vi "Ball Intake SS Implem.vi"(11 "Ball Intake Commands Out":T1) -> (3 "Ball Intake Actuator Out":T2)   [LabVIEW 2016]
uses:
  Ball Intake Actuator Out.ctl
  Ball Intake Commands.ctl
  Ball Intake Logging Values.vi
  Global Variables/Robot Status.vi
  Global Variables/Ball Intake Calibrations.vi
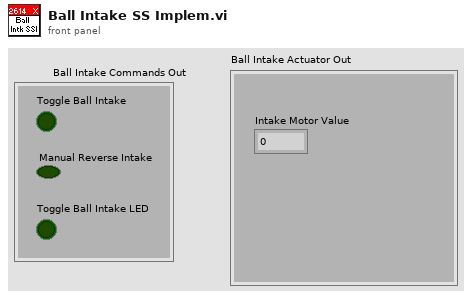
[diagram p1: front panel]
types:
  T1 = typedef "Ball Intake Commands.ctl" = cluster{"Toggle Ball Intake":bool, "Manual Reverse Intake":bool, "Toggle Ball Intake LED":bool}
  T2 = typedef "Ball Intake Actuator Out.ctl" = cluster{"Intake Motor Value":dbl}
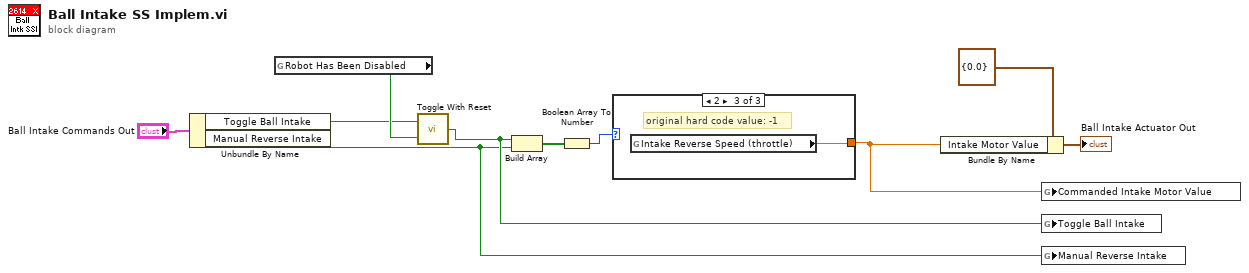
[diagram p0: block diagram]
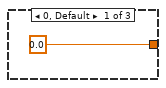
[diagram p2: hidden frame]
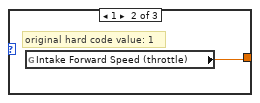
[diagram p3: hidden frame]
diagram:
  n1 = Unbundle By Name("Ball Intake Commands Out") -> ("Toggle Ball Intake"=w4:bool, "Manual Reverse Intake"=w2:bool)
  n2 = global read "Robot Status.vi" "Robot Has Been Disabled"() -> (w5:bool)
  n3 = call "Toggle With Reset.vi"("Reset"=w5, "Boolean"=w4) -> ("Driver Switch 2"=w3:bool)
  n4 = Build Array(w3, w2) -> (w7:bool[])
  n5 = Boolean Array To Number(Boolean array=w7) -> (number=w6:u32)
  n6 = case shown="2" w6 {
    tunnel: [0.0 w12 w13] -> w1
    frame 0, Default {
    }
    frame 1 {
      # "original hard code value: 1"
      n7 = global read "Ball Intake Calibrations.vi" "Intake Forward Speed (throttle)"() -> (w12:dbl)
    }
    frame 2 {
      # "original hard code value: -1"
      n8 = global read "Ball Intake Calibrations.vi" "Intake Reverse Speed (throttle)"() -> (w13:dbl)
    }
  }
  n9 = Bundle By Name(cluster=T2 {"Intake Motor Value"=0.0} ("Ball Intake Actuator Out 2"), "Intake Motor Value"=w1) -> (→"Ball Intake Actuator Out":T2)
  n10 = global write "Ball Intake Logging Values.vi" "Commanded Intake Motor Value"(w1) -> ()
  n11 = global write "Ball Intake Logging Values.vi" "Toggle Ball Intake"(w3) -> ()
  n12 = global write "Ball Intake Logging Values.vi" "Manual Reverse Intake"(w2) -> ()
